vi "Constants.vi"() -> ()   [LabVIEW 2019, in "TimingDRV Shared.lvlib"]
doc: "Use this Global VI to access the GUIDs assigned to the page resources of the Custom Device."
uses:
  TimingDRV Shared.lvlib
panel:
  in  "Tab Control":enum32{"GUIDS", "Constants", "Properties"}(tab)
  in  "Page3":string="9655e4c8-c3f0-4f2b-9b8c-78a395c1cb6e"
  in  "Page2":string="52f62866-83a2-4cd0-8a85-a9b87513a727"
  in  "Page1":string="0b83ef27-0fd3-4245-a651-6f77db6db129"
  in  "TimingDRV":string="59e4cbcc-3e84-4f48-9346-8337333d98e3"
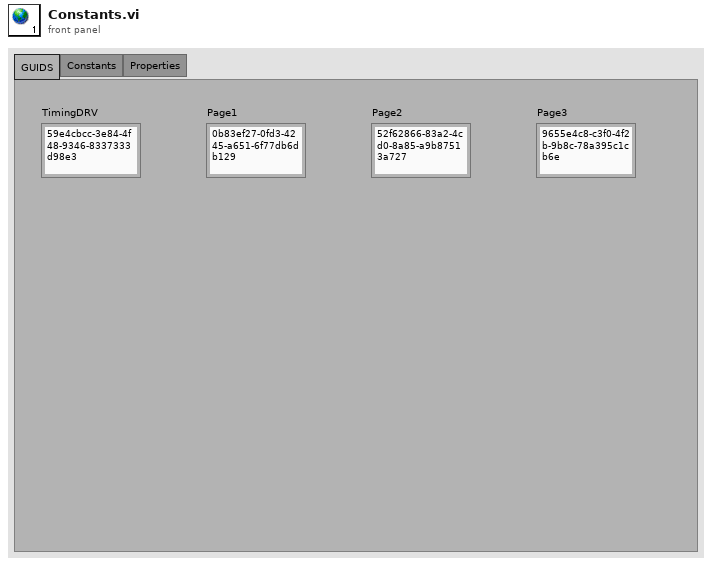
[diagram p1: front panel]
diagram:
